vi "Get Hardware Relay State.vi"(0 "DevicePropertyRelay in":refnum<class "DevicePropertyRelay.lvclass">, 5 "Session Handle in":T1, 11 "error in (no error)":errorcluster) -> (4 "DevicePropertyRelay out":refnum<class "DevicePropertyRelay.lvclass">, 10 "RelayPosition":T2=10 caption="position" items=["Open"=10, "Closed"=11], 15 "error out":errorcluster)   [LabVIEW 2015, in "SLSC Switch.lvlib" / "DevicePropertyRelay.lvclass"]
doc: "This uses a device property and/or command to get the current hardware state of a relay."
uses:
  DevicePropertyRelay.lvclass
  slscsl/RelayPosition.ctl
  SLSC Session/Typedefs/Session Handle.ctl
  SLSC Session/SLSC Session.lvclass
  DevicePropertyRelay.lvclass/DevicePropertyRelay.ctl
  slscsl/slscsl.lvclass
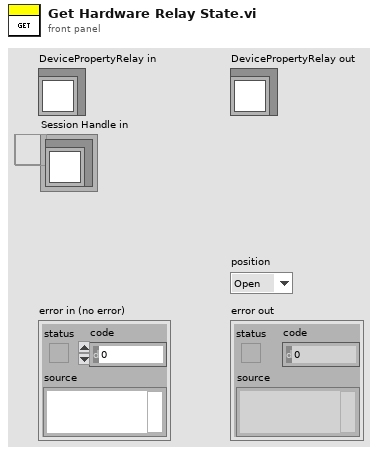
[diagram p1: front panel]
types:
  T1 = typedef "SLSC Switch.lvlib/SLSC Session.lvclass/Session Handle.ctl" = refnum<data-value>
  T2 = typedef "SLSC Switch.lvlib/slscsl.lvclass/RelayPosition.ctl" = i32
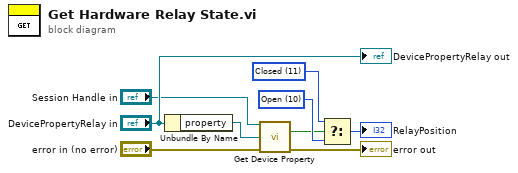
[diagram p0: block diagram]
diagram:
  w7 = T2 10 items=["Open"=10, "Closed"=11] ("f")
  w8 = T2 11 items=["Open"=10, "Closed"=11] ("RelayPosition")
  n1 = Unbundle By Name("DevicePropertyRelay in") -> ("property"=w4:refnum<k21>)
  n2 = call "Get Device Property.vi"("Session Handle in"="Session Handle in", "property"=w4, "error in (no error)"="error in (no error)") -> ("property value"=w1:bool, "error out"=→"error out":errorcluster)  [unwired: 10 in, 1 out]
  n3 = Select(t=w8, s=w1, f=w7) -> (s? t:f=→"RelayPosition":T2)
  "DevicePropertyRelay out" <- "DevicePropertyRelay in"
